vi "Add.vi"(10 "Operand 2":dbl, 11 "Operand 1":dbl) -> (3 "Numeric":dbl)   [LabVIEW 2014]
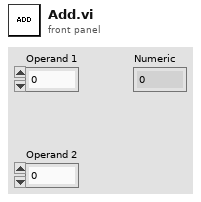
[diagram p1: front panel]
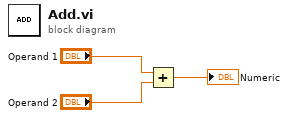
[diagram p0: block diagram]
diagram:
  n1 = Add(x="Operand 1", y="Operand 2") -> (x+y=→"Numeric":dbl)
